vi "Data to Memory.vi"(8 "error in (no error)":errorcluster, 11 "VISA resource name":refnum<visa-resource-name>) -> (0 "error out":errorcluster, 3 "VISA resource name out":refnum<visa-resource-name>)   [LabVIEW 2018, in "Agilent 87XX Series.lvlib"]
doc: "This VI for the HP8753B Network Analyzer is used to store the data trace to the channel memory. Its effect is the same as pressing the \"DATA -> MEMORY\" softkey button seen after pressing the \"DISPLAY\" button."
uses:
  Agilent 87XX Series.lvlib
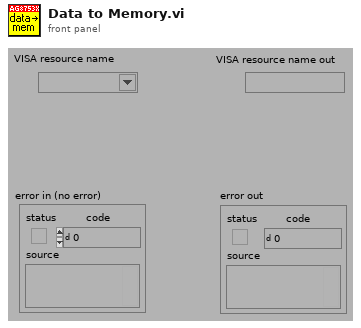
[diagram p1: front panel]
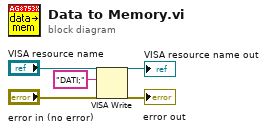
[diagram p0: block diagram]
diagram:
  n1 = VISA Write(VISA resource name="VISA resource name", write buffer="DATI;", error in (no error)="error in (no error)") -> (VISA resource name out=→"VISA resource name out":refnum<visa-resource-name>, error out=→"error out":errorcluster)  [unwired: 1 out]
